vi "ViewWindowCreate.vi"() -> (3 "SceneObject out":refnum<vi>)   [LabVIEW 2015, in "RDS Libraries.lvlib" / "lv-attitudecontrol.lvlib"]
uses:
  lv-attitudecontrol.lvlib
  Controls/PictureTypes.ctl
  <vilib>/picture/3D Picture Control/Object/Create Object (name).vi
  <vilib>/picture/3D Picture Control/NI_3D Picture Control.lvlib
panel:
  # "Generates the Viewing Window with the picture \nat the path specified below"
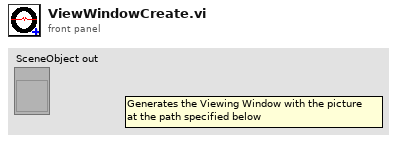
[diagram p1: front panel]
types:
  T1 = typedef "RDS Libraries.lvlib/lv-attitudecontrol.lvlib/PictureTypes.ctl" = enum16{"Fixed Horizon", "Altitude Lines", "Dial"}
  T2 = enum16{"As a Decal", "With Modulation", "With Blending", "As a replacement"}
  T3 = cluster{"Red":sgl, "Green":sgl, "Blue":sgl, "Alpha":sgl}[]
  T4 = enum16{"Overall", "Per Primitive", "Per Vertex", "Binding Off"}
  T5 = enum16{"Normal Bin", "Opaque Bin", "Transparent Bin"}
  T6 = enum16{"Points", "Lines", "Line Strip", "Line Loop", "Triangles", "Triangle Strip", "Triangle Fan", "Quads", "Quad Strip", "Polygon"}
  T7 = typedef "imagedata.ctl" = cluster{"image type":i32, "image depth":i32, "image":u8[], "mask":u8[], "colors":u32[], "Rectangle":cluster{"left":i16, "top":i16, "right":i16, "bottom":i16}}
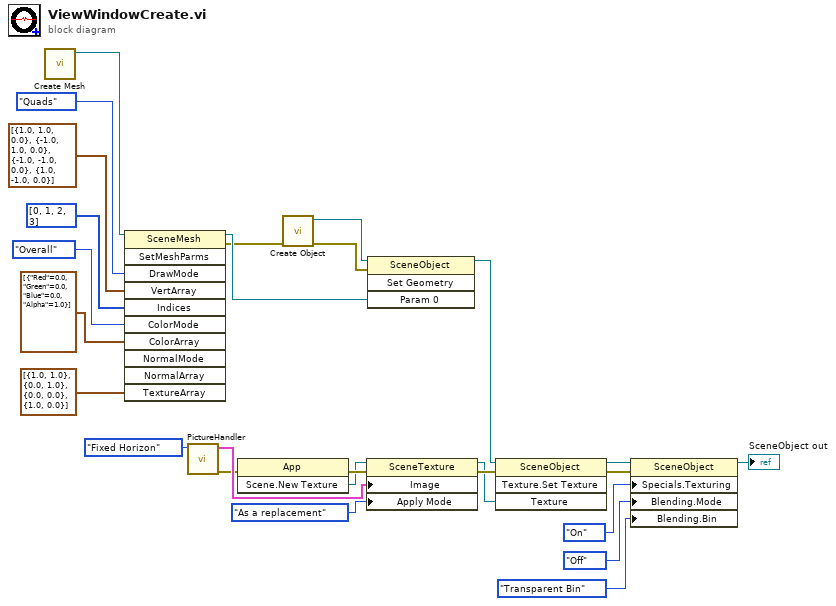
[diagram p0: block diagram]
diagram:
  n1 = call <vilib>:"Create Mesh.vi"() -> ("New Mesh Refnum"=w10:refnum<vi>)  [unwired: 10 in, 1 out]
  n2 = invoke class="SceneMesh" method="SetMeshParms"(reference=w10, "DrawMode"=T6."Quads" ("Draw Mode"), "VertArray"=cluster{"X":sgl, "Y":sgl, "Z":sgl}[] [{"X"=1.0, "Y"=1.0, "Z"=0.0}, {"X"=-1.0, "Y"=1.0, "Z"=0.0}, {"X"=-1.0, "Y"=-1.0, "Z"=0.0}, {"X"=1.0, "Y"=-1.0, "Z"=0.0}] ("Vertex Array"), "Indices"=u32[] [0, 1, 2, 3], "ColorMode"=T4."Overall" ("Color Binding Mode"), "ColorArray"=T3 [{"Red"=0.0, "Green"=0.0, "Blue"=0.0, "Alpha"=1.0}] ("Color Array"), "TextureArray"=cluster{"S":sgl, "T":sgl}[] [{"S"=1.0, "T"=1.0}, {"S"=0.0, "T"=1.0}, {"S"=0.0, "T"=0.0}, {"S"=1.0, "T"=0.0}] ("Texture Coordinate Array")) -> (reference out=w17:refnum<vi>, error out=w15:errorcluster)  [unwired: 4 in, 9 out]
  n3 = call "PictureHandler.vi"("Picture"=PictureTypes."Fixed Horizon") -> ("error out"=w1:errorcluster, "image data"=w3:T7)  [unwired: 9 in]
  n4 = invoke class="App" method="Scene.New Texture"(error in=w1) -> (error out=w8:errorcluster, "Scene.New Texture"=w7:refnum<vi>)  [unwired: 2 in, 1 out]
  n5 = call-poly <vilib>:"Create Object.vi"("error in (no error)"=w15) -> ("error out"=w16:errorcluster, "Scene:New Object"=w5:refnum<vi>)  [unwired: 9 in]
  n6 = property class="SceneTexture"(reference=w7, error in=w8, "Image"=w3, "Apply Mode"=T2."As a replacement") -> (reference out=w18:refnum<vi>, error out=w19:errorcluster)
  n7 = invoke class="SceneObject" method="Set Geometry"(reference=w5, error in=w16, "Param 0"=w17) -> (reference out=w6:refnum<vi>)  [unwired: 1 in, 3 out]
  n8 = invoke class="SceneObject" method="Texture.Set Texture"(reference=w6, error in=w19, "Texture"=w18) -> (reference out=w20:refnum<vi>, error out=w21:errorcluster)  [unwired: 1 in, 2 out]
  n9 = property class="SceneObject"(reference=w20, error in=w21, "Specials.Texturing"=enum16{"Inherit Value", "Off", "On"}."On" ("Specials:Texturing"), "Blending.Mode"=enum16{"Inherit Value", "Off", "On"}."Off" ("Blending:Mode 2"), "Blending.Bin"=T5."Transparent Bin" ("Blending:Bin")) -> (reference out=→"SceneObject out":refnum<vi>)  [unwired: 1 out]
